vi "FGV.vi"(5 "Enum":enum16{"Write", "Read"}(ring)=enum."Read", 9 "IN":T1={"Play"=FALSE, "rate"=1000.0, "samples per channel"=1000} {"rate" format="%0.2f"}) -> (2 "OUT":T1={"Play"=FALSE, "rate"=1000.0, "samples per channel"=1000} {"rate" format="%0.2f"})   [LabVIEW 2016]
uses:
  Typedefs/FGV_params.ctl
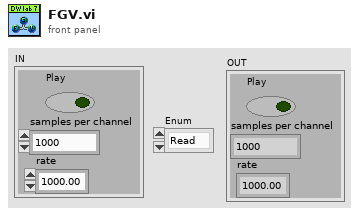
[diagram p1: front panel]
types:
  T1 = typedef "FGV_params.ctl" = cluster{"Play":bool, "rate":dbl, "samples per channel":i32}
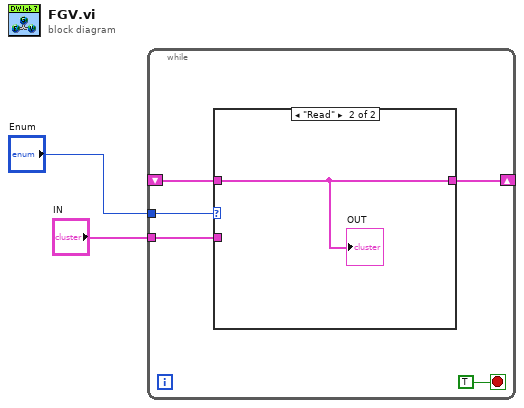
[diagram p0: block diagram]
diagram:
  n1 = while {
    tunnel: "IN" -> [w6]
    shift-right: [w5] -> _
    shift-left: _ -> [w4]
    tunnel: "Enum" -> [w3]
    stop <- TRUE stop-if-true
    n2 = case shown="\"Read\"" w3 {
      tunnel: w6 -> [w8 _]
      tunnel: [w8 w9] -> w5
      tunnel: w4 -> [_ w9]
      frame "Write", Default {
      }
      frame "Read" {
        "OUT" <- w9
      }
    }
  }
